vi "Strip Out Owning Libraries.vi"(1 "Original Name":string) -> (0 "Name w/o Libraries":string)   [LabVIEW 2016, in "Flex UI.lvclass"]
uses:
  Flex UI.lvclass
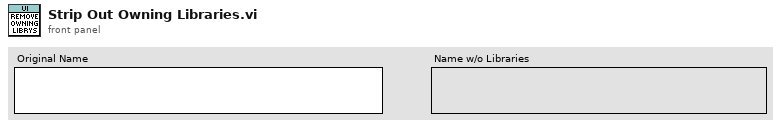
[diagram p1: front panel]
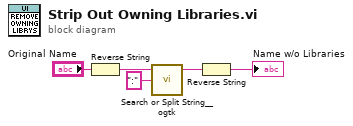
[diagram p0: block diagram]
diagram:
  n1 = Reverse String(1:"Original Name") -> (0:w4:string)
  n2 = call <userlib>:"Search or Split String__ogtk.vi"("search string/char (-)"=":", "string"=w4) -> ("substring before match"=w2:string)  [unwired: 1 in, 2 out]
  n3 = Reverse String(1:w2) -> (0:→"Name w/o Libraries":string)
